vi "Reset.vi"(8 "error in (no error)":errorcluster, 11 "SLSC Switch in":refnum<class "SLSC Switch.lvclass">) -> (0 "error out":errorcluster, 3 "SLSC Switch out":refnum<class "SLSC Switch.lvclass">)   [LabVIEW 2016, in "SLSC Switch.lvlib" / "SLSC Switch.lvclass"]
doc: "Opens all relays."
uses:
  SLSC Switch.lvclass
  Controls/Connection.ctl
  slscsl/RelayAction.ctl
  SLSC Switch.lvclass/SLSC Switch.ctl
  Relay/Relay.lvclass/Relay.ctl
  Relay/Read relay name.vi
  <vilib>/SLSC/Flatten Names (String).vi
  Switch Action Processor/Switch Action Processor.lvclass
  <vilib>/SLSC/SLSC.lvlib
  slscsl/slscsl.lvclass
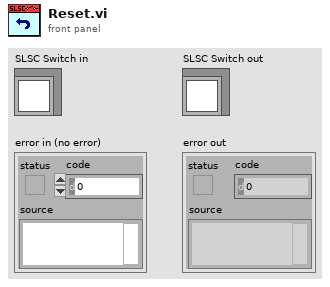
[diagram p1: front panel]
types:
  T1 = typedef "SLSC Switch.lvlib/SLSC Switch.lvclass/Connection.ctl" = cluster{"channel 1":string, "channel 2":string}
  T2 = typedef "SLSC Switch.lvlib/slscsl.lvclass/RelayAction.ctl" = u32
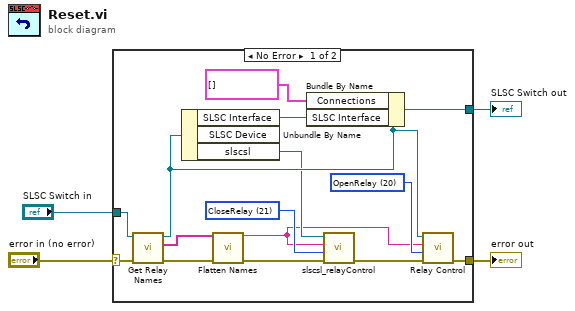
[diagram p0: block diagram]
diagram:
  n1 = case shown="No Error" "error in (no error)" {
    selector: "error in (no error)" -> [w15 w21]
    tunnel: [w12 w21] -> w3
    tunnel: [w17 w20] -> w1
    tunnel: "SLSC Switch in" -> [w19 w20]
    frame No Error {
      w6 = T2 21 items=["CloseRelay"=21, "OpenRelay"=20] ("RelayAction")
      w10 = T2 20 items=["CloseRelay"=21, "OpenRelay"=20] ("relay action")
      n2 = call "Get Relay Names.vi"("error in (no error)"=w15, "SLSC Switch in"=w19) -> ("error out"=w14:errorcluster, "Relay Names"=w16:string[], "SLSC Switch out"=w11:refnum<class "SLSC Switch.lvclass">)  [unwired: 7 in]
      n3 = Unbundle By Name(w11) -> ("SLSC Interface"=w13:refnum<class "SLSC Interface.lvclass">, "slscsl"=w7:refnum<class "slscsl.lvclass">)  [unwired: 1 out]
      n4 = call-poly <vilib>:"Flatten Names.vi"("names in"=w16, "error in (no error)"=w14) -> ("names out"=w5:string, "error out"=w9:errorcluster)  [unwired: 12 in]
      n5 = Bundle By Name(cluster=w11, "Connections"=T1[] [], "SLSC Interface"=w13) -> (w17:refnum<class "SLSC Switch.lvclass">)
      n6 = call "slscsl_relayControl.vi"("error in (no error)"=w9, "RelayAction"=w6, "relayNames"=w5, "slscsl in"=w7) -> ("error out"=w8:errorcluster)  [unwired: 5 in, 2 out]
      n7 = call "Relay Control.vi"("error in (no error)"=w8, "relay action"=w10, "relay names"=w5, "SLSC Switch in"=w11) -> ("error out"=w12:errorcluster)  [unwired: 6 in, 1 out]
    }
    frame Error {
    }
  }
  "error out" <- w3
  "SLSC Switch out" <- w1
